vi "Abort Structure.vi"(0 "Abort Constant In":bool, 1 "Processed Data Notifier":refnum<notifier>, 2 "Abort Parameters":T2 {"Abort Criteria"."Comparison" items=["<", ">"]}, 3 "Calibration Configuration":T1, 11 "Clock timer (s)":dbl, 12 "error in":errorcluster) -> (4 "Abort Constant Out":bool, 14 "error out":errorcluster, 15 "Status":string)   [LabVIEW 2024]
uses:
  Abort Parameters.ctl
  Configuration/Calibration Configuration.ctl
  support/Control/Array Data Constant.ctl
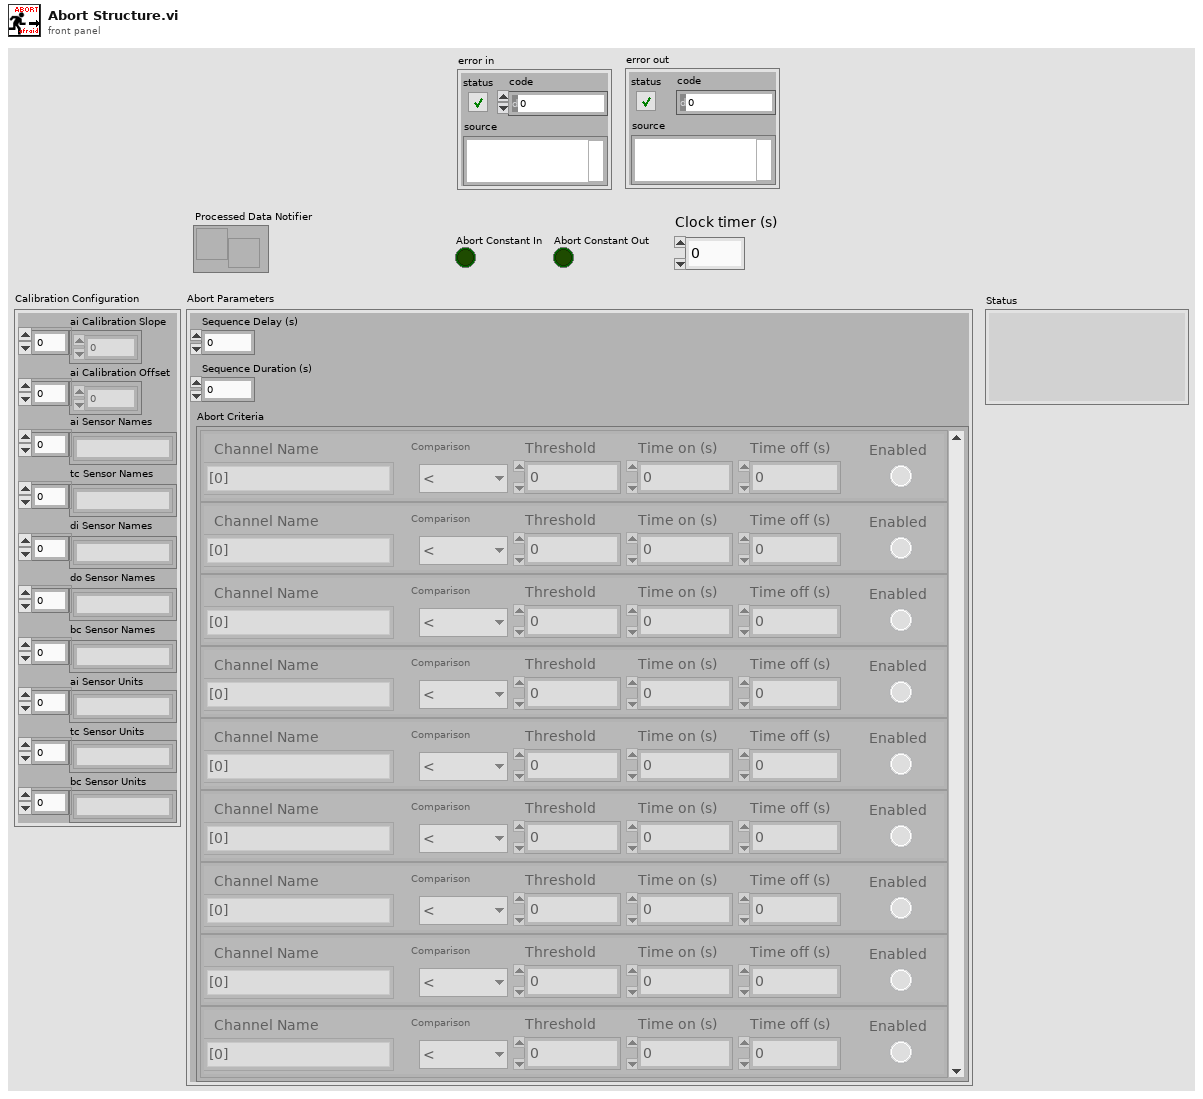
[diagram p1: front panel]
types:
  T1 = typedef "Calibration Configuration.ctl" = cluster{"ai Calibration Slope":dbl[], "ai Calibration Offset":dbl[], "ai Sensor Names ":string[], "tc Sensor Names":string[], "di Sensor Names":string[], "do Sensor Names":string[], "bc Sensor Names":string[], "ai Sensor Units":string[], "tc Sensor Units":string[], "bc Sensor Units":string[]}
  T2 = typedef "Abort Parameters.ctl" = cluster{"Sequence Delay (s)":dbl, "Sequence Duration (s)":dbl, "Abort Criteria":cluster{"Channel Name\n":enum16{"[0]", "[1]", "[2]", "[3]", "[4]", "[5]", "[6]", "[7]", "[8]", "[9]", "[10]", "[11]", "[12]", "[13]", "[14]", "[15]", "[16]", "[17]", "[18]", "[19]", "[20]", "[21]", "[22]", "[23]", "[24]", "[25]", "[26]", "[27]", "[28]", "[29]", "[30]", "[31]", "[32]", "[33]", "[34]", "[35]", "[36]", "[37]", "[38]", "[39]", "[40]", "[41]", "[42]", "[43]", "[44]", "[45]", "[46]", "[47]", "[48]", "[49]"}, "Comparison\n":u16, "Threshold":dbl, "Time on (s)":dbl, "Time off (s)":dbl, "Enabled":bool}[]}
  T3 = cluster{"Channel Name\n":enum16{"[0]", "[1]", "[2]", "[3]", "[4]", "[5]", "[6]", "[7]", "[8]", "[9]", "[10]", "[11]", "[12]", "[13]", "[14]", "[15]", "[16]", "[17]", "[18]", "[19]", "[20]", "[21]", "[22]", "[23]", "[24]", "[25]", "[26]", "[27]", "[28]", "[29]", "[30]", "[31]", "[32]", "[33]", "[34]", "[35]", "[36]", "[37]", "[38]", "[39]", "[40]", "[41]", "[42]", "[43]", "[44]", "[45]", "[46]", "[47]", "[48]", "[49]"}, "Comparison\n":u16, "Threshold":dbl, "Time on (s)":dbl, "Time off (s)":dbl, "Enabled":bool}[]
  T4 = typedef "Array Data Constant.ctl" = cluster{"AI":dbl[], "TC":dbl[], "BC":dbl[], "DI":dbl[], "t (UTC)":dbl}
  T5 = enum16{"[0]", "[1]", "[2]", "[3]", "[4]", "[5]", "[6]", "[7]", "[8]", "[9]", "[10]", "[11]", "[12]", "[13]", "[14]", "[15]", "[16]", "[17]", "[18]", "[19]", "[20]", "[21]", "[22]", "[23]", "[24]", "[25]", "[26]", "[27]", "[28]", "[29]", "[30]", "[31]", "[32]", "[33]", "[34]", "[35]", "[36]", "[37]", "[38]", "[39]", "[40]", "[41]", "[42]", "[43]", "[44]", "[45]", "[46]", "[47]", "[48]", "[49]"}
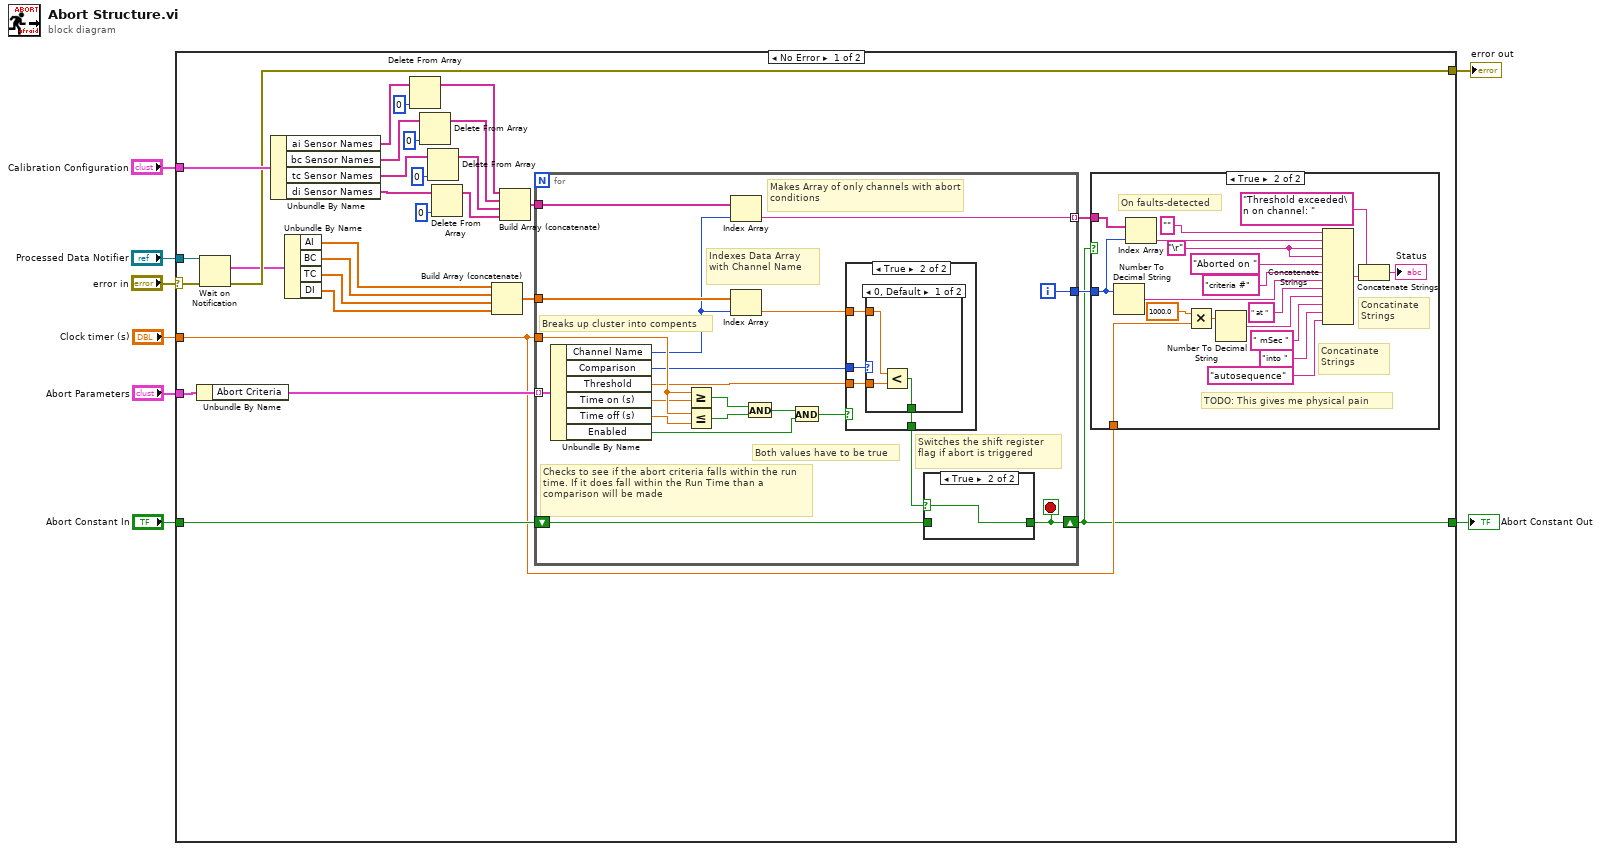
[diagram p0: block diagram]
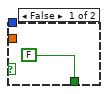
[diagram p3: hidden frame]
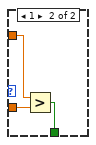
[diagram p4: hidden frame]
diagram:
  n1 = case shown="No Error" "error in" {
    selector: "error in" -> [w18 w92]
    tunnel: "Abort Constant In" -> [w38 w91]
    tunnel: "Abort Parameters" -> [w33 _]
    tunnel: "Processed Data Notifier" -> [w16 _]
    tunnel: "Clock timer (s)" -> [w31 _]
    tunnel: [w17 w92] -> w4
    tunnel: "Calibration Configuration" -> [w34 _]
    tunnel: [w9 w91] -> w1
    frame No Error {
      n2 = Unbundle By Name(w33) -> ("Abort Criteria"=w35:T3)
      n3 = Wait on Notification(notifier=w16, error in (no error)=w18) -> (notification=w15:T4, error out=w17:errorcluster)  [unwired: 2 in, 2 out]
      n4 = Unbundle By Name(w34) -> ("ai Sensor Names"=w30:string[], "bc Sensor Names"=w26:string[], "tc Sensor Names"=w24:string[], "di Sensor Names"=w22:string[])
      n5 = Unbundle By Name(w15) -> ("AI"=w13:dbl[], "BC"=w12:dbl[], "TC"=w11:dbl[], "DI"=w10:dbl[])
      n6 = Delete From Array(array=w30, index=0) -> (array with subset deleted=w29:string[])  [unwired: 1 in, 1 out]
      n7 = Delete From Array(array=w26, index=0) -> (array with subset deleted=w21:string[])  [unwired: 1 in, 1 out]
      n8 = Delete From Array(array=w24, index=0) -> (array with subset deleted=w20:string[])  [unwired: 1 in, 1 out]
      n9 = Delete From Array(array=w22, index=0) -> (array with subset deleted=w19:string[])  [unwired: 1 in, 1 out]
      n10 = Build Array (concatenate)(w13, w12, w11, w10) -> (w14:dbl[])
      n11 = Build Array (concatenate)(w29, w21, w20, w19) -> (w32:string[])
      n12 = for {
        tunnel: w35 -> [w50] mode=indexing
        tunnel: w14 -> [w58]
        shift-right: [w41] -> w9
        shift-left: w38 -> [w51]
        tunnel: w31 -> [w53]
        tunnel: w32 -> [w55]
        tunnel: [w54] -> w36 mode=indexing
        tunnel: [w40] -> w37
        i -> [w40]
        stop <- w41 stop-if-true
        # "Breaks up cluster into compents"
        # "Makes Array of only channels with abort conditions"
        # "Switches the shift register flag if abort is triggered"
        # "Both values have to be true"
        # "Indexes Data Array with Channel Name"
        # "Checks to see if the abort criteria falls within the run time. If it does fall within the Run Time than a comparison will be made"
        n13 = Unbundle By Name(w50) -> ("Channel Name"=w49:T5, "Comparison"=w47:u16, "Threshold"=w46:dbl, "Time on (s)"=w45:dbl, "Time off (s)"=w39:dbl, "Enabled"=w42:bool)
        n14 = Greater Or Equal?(x=w53, y=w45) -> (x >= y?=w48:bool)
        n15 = Less Or Equal?(x=w53, y=w39) -> (x <= y?=w57:bool)
        n16 = Index Array(array=w55, index=w49) -> (element=w54:string)
        n17 = Index Array(array=w58, index=w49) -> (element=w56:dbl)
        n18 = And(x=w48, y=w57) -> (x .and. y?=w43:bool)
        n19 = And(x=w43, y=w42) -> (x .and. y?=w44:bool)
        n20 = case shown="True" w44 {
          tunnel: w47 -> [_ w65]
          tunnel: w56 -> [_ w64]
          tunnel: [FALSE ("Blank Button 3") w63] -> w52
          tunnel: w46 -> [_ w62]
          frame False {
          }
          frame True {
            n21 = case shown="0, Default" w65 {
              tunnel: w64 -> [w68 w71]
              tunnel: [w67 w70] -> w63
              tunnel: w62 -> [w66 w69]
              frame 0, Default {
                n22 = Less?(x=w68, y=w66) -> (x < y?=w67:bool)
              }
              frame 1 {
                n23 = Greater?(x=w71, y=w69) -> (0:w70:bool)
              }
            }
          }
        }
        n24 = case shown="True" w52 {
          selector: w52 -> [_ w60]
          tunnel: [w59 w60] -> w41
          tunnel: w51 -> [w59 _]
          frame False {
          }
          frame True {
          }
        }
      }
      n25 = case shown="True" w9 {
        tunnel: w36 -> [_ w90]
        tunnel: w31 -> [_ w73]
        tunnel: w37 -> [_ w82]
        frame False {
        }
        frame True {
          w78 = "\r"
          # "TODO: This gives me physical pain"
          # "Concatinate \nStrings"
          # "Concatinate \nStrings"
          # "On faults-detected"
          n26 = Number To Decimal String(number=w82) -> (decimal integer string=w84:string)  [unwired: 1 out]
          n27 = Index Array(array=w90, index=w82) -> (element=w85:string)
          n28 = Multiply(x=1000.0, y=w73) -> (x*y=w74:dbl)
          n29 = Number To Decimal String(number=w74) -> (decimal integer string=w83:string)  [unwired: 1 out]
          n30 = Concatenate Strings("", w85, w78, w78, "Aborted on ", "criteria #", w84, " at ", w83, " mSec ", "into ", "autosequence") -> (w87:string)
          n31 = Concatenate Strings("Threshold exceeded\n on channel: ", w87) -> (→"Status":string)
        }
      }
    }
    frame Error {
    }
  }
  "error out" <- w4
  "Abort Constant Out" <- w1
